vi "例9.5 利用声卡输出波形.vi"() -> ()   [LabVIEW 2012]
doc: "本VI说明了生成并播放正弦波、方波、锯齿波和三角波的方式。在连续播放时可更改生成波形的频率和类型。"
uses:
  <vilib>/sound2/lvsound2.llb/Sampling Mode.ctl
  <vilib>/sound2/lvsound2.llb/Sound Output Set Volume (Single).vi
  <vilib>/sound2/lvsound2.llb/Sound Output Write (DBL Single).vi
  <vilib>/measure/NI_MABase.lvlib
panel:
  in  "声音格式":cluster{"采样率":dbl, "通道数":dbl, "每采样比特数":dbl}={"采样率"=44100.0, "通道数"=2.0, "每采样比特数"=16.0}
  in  "声音大小":dbl(slide)=70.40816326530613 caption="音量" scale=0.0..100.0
  out "产生的声音波形":waveform(dbl)(graph) caption="生成声音"
  in  "频率":dbl=500.0 format="%0.2p"
  in  "Number of Samples/ch":i32=5000 caption="每通道采样数"
  in  "Device ID":u32 caption="设备ID"
  # "本VI说明了生成并连续播放正弦波、方波、锯齿波和三角波的方式。\n\n执行VI步骤：\n1.  指定设备ID、每采样比特数、采样率和采样数（缓冲区大小）。\n2.  选择需播放的波形类型以及初始频率。\n3.  运行VI。将生成波形并发送至图形和扬声器。\n3.  更改频率可改变声音的音调。\n4.  更改波形类型可开始播放其它波形。\n5.  完成时按停止按钮。"
  # "配置"
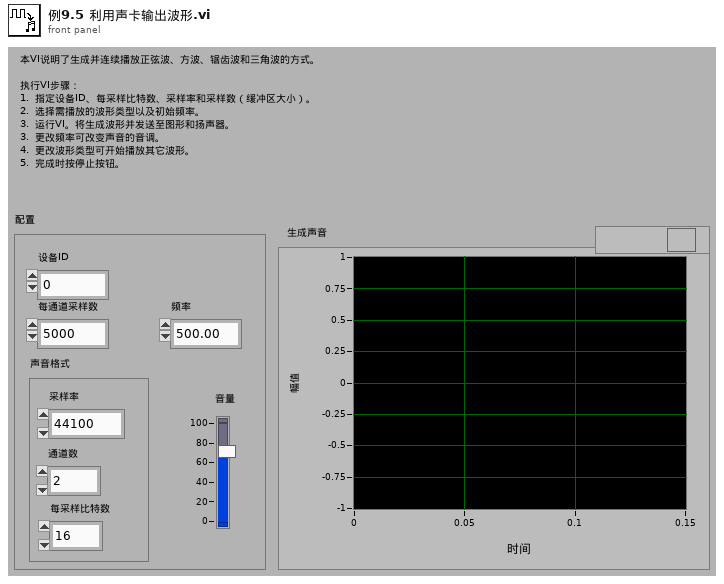
[diagram p1: front panel]
types:
  T1 = typedef "Sampling Mode.ctl" = i32
  T2 = typedef "Sound Output Task ID.ctl" = u32
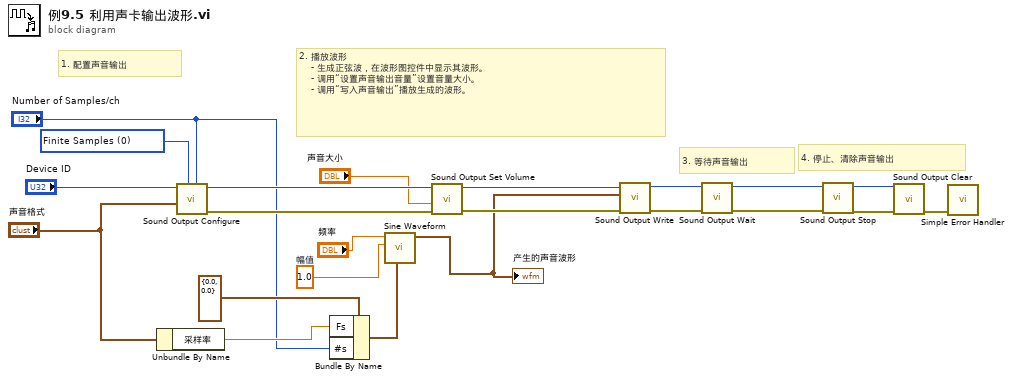
[diagram p0: block diagram]
diagram:
  w15 = 1.0  # 幅值
  w19 = T1 0 items=["Finite Samples", "Continuous Samples"] ("sample mode")
  # "3. 等待声音输出"
  # "4. 停止、清除声音输出"
  # "2. 播放波形\n\t   - 生成正弦波，在波形图控件中显示其波形。\n    - 调用“设置声音输出音量”设置音量大小。\n    - 调用“写入声音输出”播放生成的波形。"
  # "1. 配置声音输出"
  n1 = Unbundle By Name("声音格式") -> ("采样率"=w10:dbl)
  n2 = call <vilib>:"Sound Output Configure.vi"("number of samples/ch"="Number of Samples/ch", "sample mode"=w19, "sound format"="声音格式", "device ID"="Device ID") -> ("error out"=w22:errorcluster, "task ID"=w21:T2)  [unwired: 6 in]
  n3 = Bundle By Name(cluster=cluster{"Fs":dbl, "#s":dbl} {"Fs"=0.0, "#s"=0.0} ("sampling info"), "Fs"=w10, "#s"="Number of Samples/ch") -> (w17:cluster{"Fs":dbl, "#s":dbl})
  n4 = call <vilib>:"Sine Waveform.vi"("sampling info"=w17, "amplitude"=w15, "frequency"="频率") -> ("signal out"=w1:waveform(dbl))  [unwired: 7 in, 1 out]
  "产生的声音波形" <- w1
  n5 = call-poly <vilib>:"Sound Output Set Volume.vi"("error in (no error)"=w22, "volume"="声音大小", "task ID"=w21) -> ("error out"=w14:errorcluster, "task ID out"=w13:T2)  [unwired: 7 in]
  n6 = call-poly <vilib>:"Sound Output Write.vi"("error in (no error)"=w14, "data"=w1, "task ID"=w13) -> ("error out"=w6:errorcluster, "task ID out"=w7:T2)  [unwired: 7 in]
  n7 = call <vilib>:"Sound Output Wait.vi"("error in (no error)"=w6, "task ID"=w7) -> ("error out"=w4:errorcluster, "task ID out"=w5:T2)  [unwired: 8 in]
  n8 = call <vilib>:"Sound Output Stop.vi"("error in (no error)"=w4, "task ID"=w5) -> ("error out"=w8:errorcluster, "task ID out"=w9:T2)  [unwired: 8 in]
  n9 = call <vilib>:"Sound Output Clear.vi"("error in (no error)"=w8, "task ID"=w9) -> ("error out"=w16:errorcluster)  [unwired: 9 in]
  n10 = call <vilib>:"Simple Error Handler.vi"("error in (no error)"=w16) -> ()  [unwired: 4 in, 5 out]
